vi "Setup Timer 1.vi"(8 "error in (no error)":errorcluster, 9 "Count (-1)":i32=-1, 10 "Period":i32, 11 "Run(T)":bool=TRUE) -> (0 "error out":errorcluster)   [LabVIEW 2015, in "Tool Module.lvlib"]
uses:
  Tool Module.lvlib
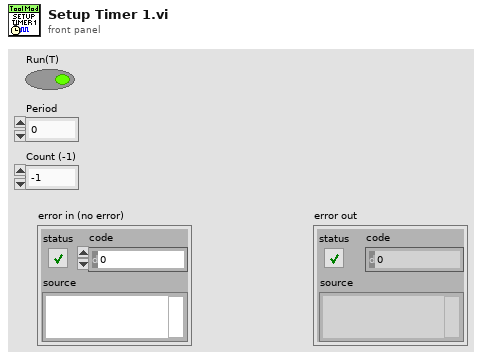
[diagram p1: front panel]
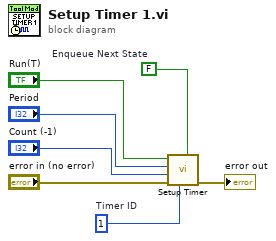
[diagram p0: block diagram]
diagram:
  w1 = 1  # Timer ID
  w7 = FALSE  # Enqueue Next State
  n1 = call "Setup Timer.vi"("Enqueue Next State"=w7, "Timer ID"=w1, "error in (no error)"="error in (no error)", "Count"="Count (-1)", "Period"="Period", "Timer On"="Run(T)") -> ("error out"=→"error out":errorcluster)  [unwired: 5 in]
